vi "Bundle Script_Invoke Node Method Change.vi"(8 "error in":errorcluster, 10 "Property Array":T2(array[cluster]), 11 "Affected Items":T1) -> (0 "error out":errorcluster, 2 "Objects":refnum<vi>[](array[refnum]))   [LabVIEW 2023]
uses:
  top/BundleMagic.ctl
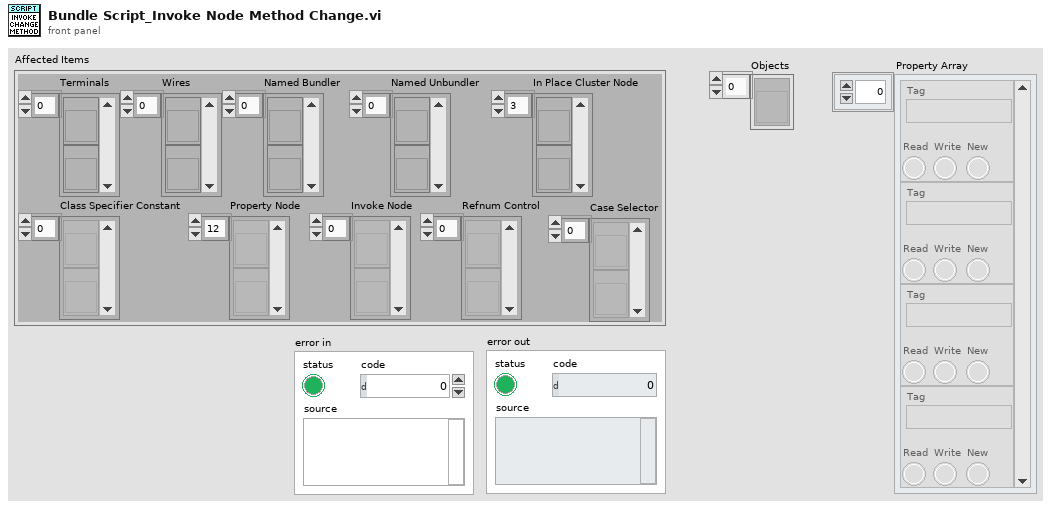
[diagram p1: front panel]
types:
  T1 = typedef "BundleMagic.ctl" = cluster{"Terminals":refnum<vi>[], "Wires":refnum<vi>[], "Named Bundler":refnum<vi>[], "Named Unbundler":refnum<vi>[], "In Place Cluster Node":refnum<vi>[], "Class Specifier Constant":refnum<vi>[], "Property Node":refnum<vi>[], "Invoke Node":refnum<vi>[], "Refnum Control":refnum<vi>[], "Case Selector":refnum<vi>[]}
  T2 = cluster{"Tag":string, "Read":bool, "Write":bool, "New":bool}[]
  T3 = cluster{"Tag":string, "Read":bool, "Write":bool, "New":bool}
  T4 = cluster{"Index":u16, "Property Type":enum16{"Unknown", "Base", "Scripting", "Private", "Deprecated", "None", "Divider"}, "ID String":string, "Dotted ID String":string, "Class":string, "Parent":string, "Display name full":string, "Display name short":string, "Parents Array":string[], "Indent":u16}
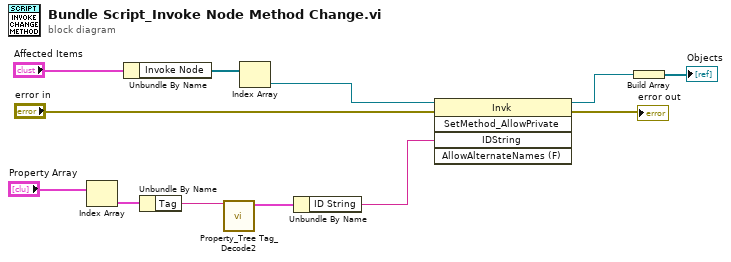
[diagram p0: block diagram]
diagram:
  n1 = Index Array(array="Property Array") -> (element=w9:T3)  [unwired: 1 in]
  n2 = Unbundle By Name("Affected Items") -> ("Invoke Node"=w12:refnum<vi>[])
  n3 = Unbundle By Name(w9) -> ("Tag"=w3:string)
  n4 = call "Property_Tree Tag_Decode2.vi"("Tag In"=w3) -> ("TagData"=w2:T4)  [unwired: 10 in]
  n5 = Index Array(array=w12) -> (element=w7:refnum<vi>)  [unwired: 1 in]
  n6 = Unbundle By Name(w2) -> ("ID String"=w1:string)
  n7 = invoke class="Invk" method="SetMethod_AllowPrivate"(reference=w7, error in="error in", "IDString"=w1) -> (reference out=w6:refnum<vi>, error out=→"error out":errorcluster)  [unwired: 2 in, 3 out]
  n8 = Build Array(w6) -> (→"Objects":refnum<vi>[])
